vi "Message Queue Reference Functional Global Variable.vi"(8 "Error In":errorcluster, 10 "Operation":T1, 11 "Message Queue Reference In":T2) -> (0 "Error Out":errorcluster, 3 "Message Queue Reference Out":T2)   [LabVIEW 2023, in "QSM - Security.lvlib"]
doc: "This VI is the message queue reference functional global variable for the Queued State Machine template."
uses:
  QSM - Security.lvlib
  Controls/Message Queue Reference.ctl
  Controls/Message Queue Element.ctl
  Controls/State Machine Message.ctl
  Controls/Message Queue Reference Functional Global Variable Operation.ctl
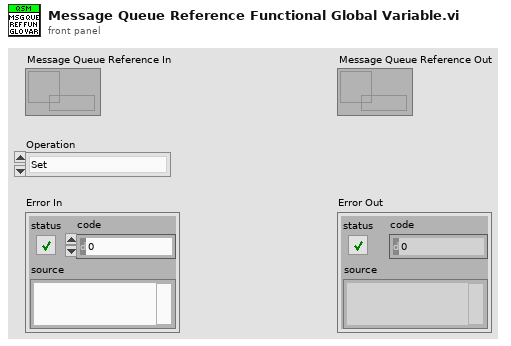
[diagram p1: front panel]
types:
  T1 = typedef "QSM - Security.lvlib/Message Queue Reference Functional Global Variable Operation.ctl" = enum16{"Set", "Get"}
  T2 = typedef "QSM - Security.lvlib/Message Queue Reference.ctl" = refnum<queue>
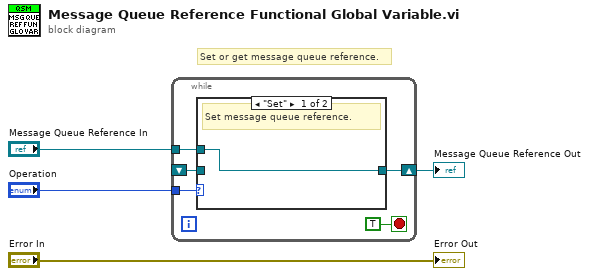
[diagram p0: block diagram]
diagram:
  # "Set or get message queue reference."
  n1 = while {
    shift-right: [w7] -> w1
    shift-left: _ -> [w6]
    tunnel: "Operation" -> [w9]
    tunnel: "Message Queue Reference In" -> [w8]
    stop <- TRUE stop-if-true
    n2 = case shown="\"Set\"" w9 {
      tunnel: w8 -> [w10 _]
      tunnel: [w10 w11] -> w7
      tunnel: w6 -> [_ w11]
      frame "Set" {
        # "Set message queue reference."
      }
      frame "Get" {
        # "Get message queue reference."
      }
    }
  }
  "Message Queue Reference Out" <- w1
  "Error Out" <- "Error In"
